vi "Project Path.vi"(8 "error in (no error)":errorcluster, 9 "Operation":enum16{"Get", "Set"}(ring), 11 "Path":path) -> (0 "error out":errorcluster, 3 "Path (out)":path)   [LabVIEW 2017, in "WebServiceImporter.lvlib" / "VI Generator.lvlib"]
uses:
  <vilib>/Platform/WebService/VI Generator/VI Generator.lvlib
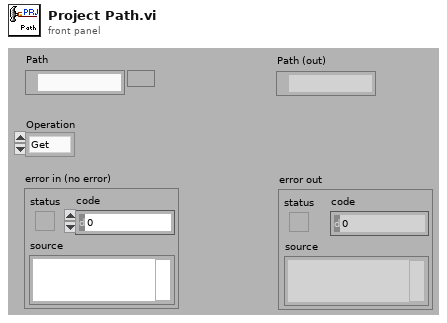
[diagram p1: front panel]
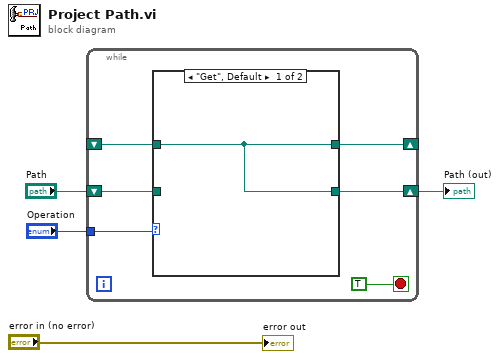
[diagram p0: block diagram]
diagram:
  n1 = while {
    tunnel: "Operation" -> [w9]
    shift-right: [w7] -> w1
    shift-left: "Path" -> [w8]
    shift-right: [w6] -> _
    shift-left: _ -> [w5]
    stop <- TRUE stop-if-true
    n2 = case shown="\"Get\", Default" w9 {
      tunnel: w8 -> [_ w12]
      tunnel: [w11 w12] -> w7
      tunnel: [w11 w12] -> w6
      tunnel: w5 -> [w11 _]
      frame "Get", Default {
      }
      frame "Set" {
      }
    }
  }
  "Path (out)" <- w1
  "error out" <- "error in (no error)"
